vi "Get Analog Vars.vi"(0 "Common alarm handling(F)":bool, 7 "Tool":bool, 11 "error in (no error)":errorcluster) -> (4 "Catagorised  Stsaus":T1[](array[typedef]), 6 "Values":dbl[](array[numeric]), 8 "Analog Vars":T4[](array[typedef]) {"Value" format="%#.1f"}, 10 "Any Alarm":bool, 13 "Primary Action":T3, 14 "Alarms":bool[](array[boolean]), 15 "error out":errorcluster)   [LabVIEW 2011]
uses:
  GUI/Analog Var Disp 0 sif.ctl
  GUI/Status indicator Black Small.ctl
  Action List.ctl
  Catagorised alarm state.ctl
  GUI/Status Indikator Helper.ctl
  Common/Variable List Common Analog.ctl
  Tool/Variable List Tool Analog.ctl
  Action Analog Handler.ctl
  <vilib>/Utility/VariantDataType/GetNumericInfo.vi
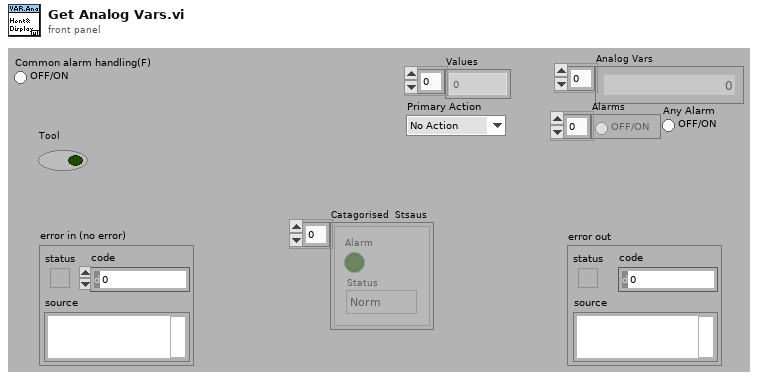
[diagram p1: front panel]
types:
  T1 = typedef "Catagorised alarm state.ctl" = cluster{"Alarm":bool, "Status":T2}
  T2 = typedef "Status Indikator Helper.ctl" = enum16{"Norm", "L", "H", "LL", "HH", "Value", "Technical"}
  T3 = typedef "Action List.ctl" = enum16{"No Action", "Stop Motor", "Turn Off HV"}
  T4 = typedef "Analog Var Disp 0 sif.ctl" = cluster{"Value":dbl, "Unit":string, "Status":T5}
  T5 = typedef "Status indicator Black Small.ctl" = u16
  T6 = typedef "Variable List Tool Analog.ctl" = enum16{"Tool Max Temperature", "Tool (Controller) Temperature", "Tool Supply Voltage", "Tool (Controller) Current", "Tool Acceleration X", "Tool Acceleration Y", "Tool Acceleration Z", "Tool Acceleration Sum", "Tool Inclination", "Tool Rotation", "Tool GP Sensor 1", "Tool GP Sensor 2", "Tool (Pressure 1) Temperature", "Tool Pressure 1 RAW", "Tool (Pressure 2) Temperature", "Tool Pressure 2 RAW", "Tool (Solenoid) Temperature", "Tool Solenoid Position", "PSU Temp", "Head Voltage", "PSU Main Voltage out", "PSU Main Current out", "Upper Tension Sub Temp", "Tool Upper Tension Sub Raw", "Lower Tension Sub Temp", "Tool Lower Tension Sub Raw", "Tool Var27 - Reserved", "Tool Var28 - Reserved", "Tool Var29 - Reserved", "Tool Var30 - Reserved", "Stroke Extension", "Stroke In Force", "Stroke Out Force", "Stroke Force", "Stroker Pressure 1", "Stroker Pressure 2", "Stroker Upper Tension Sub", "Stroker Lower Tension Sub", "Stroker Var09 - Reserved", "Stroker Var10 - Reserved", "Tractor Upper Tension Sub", "Tractor Lower Tension Sub", "Tractor Var03 - Reserved", "Tractor Var04 - Reserved", "Tool Temperature sensor", "Tool Motor Voltage", "Tool Motor Current", "Tool Motor Torque", "Tool weight on bit", "Tool Motor RPM"}
  T7 = typedef "Variable List Common Analog.ctl" = enum16{"HVPSU Head Voltage", "HVPSU TS Voltage", "HVPSU Current", "PCP Cable Resistance", "Winch Depth", "Winch Line Speed", "Winch Wire Tension"}
  T8 = typedef "Action Analog Handler.ctl" = enum16{"GET value", "GET Single Frequenzy", "GET All Values", "GET Waveform", "Get Numb Var", "SET Value", "START Buffer", "REG Variable", "BUF size(total antal sekund)", "PULS", "Get a Value at time", "Set initial waveform"}
  T9 = typedef "User Setting Analog Channel Bg.ctl" = cluster{"Scaling":T10, "Limits and responces":T11, "Allow Graph selection by user":bool, "Unit":u16}
  T10 = typedef "Scaling.ctl" = cluster{"Gain":dbl, "Offset":dbl}
  T11 = typedef "Alarm Setup Analog.ctl" = cluster{"Technical Error(NA)":T12, "LL":T12, "L":T12, "H":T12, "HH":T12, "Limits":T13}
  T12 = typedef "Alarm Responce.ctl" = cluster{"Action":T3, "Alarm":bool}
  T13 = typedef "Limits.ctl" = cluster{"LL":dbl, "L":dbl, "H":dbl, "HH":dbl}
  T14 = typedef "Fixed Analog Channel Definition.ctl" = cluster{"ID":u16, "Name":string, "Quantity":T15, "Unit":string, "Maximum upd":T16, "Comment":string, "Help file Name":string, "Help file Section ":string, "Category":T17, "User adjustable Scaling":bool, "Default Scaling":T10, "Default Unit":i32, "Classification":T18}
  T15 = typedef "Quantity enum.ctl" = enum16{"NA", "Acceleration", "Angle", "Current", "Force", "Distance", "Pressure", "Resistance", "Rotational Speed", "Speed", "Temperature", "Tension", "Torque", "Voltage", "Weight"}
  T16 = typedef "Update frequensies.ctl" = enum16{"2 Hz", "1 Hz", "0.1 Hz"}
  T17 = typedef "Channel catagory Enum.ctl" = enum16{"No Category", "Power", "Temperature", "Pressure"}
  T18 = typedef "Channel Classification Enum.ctl" = enum16{"Basic", "Advanced", "Expert", "Unused"}
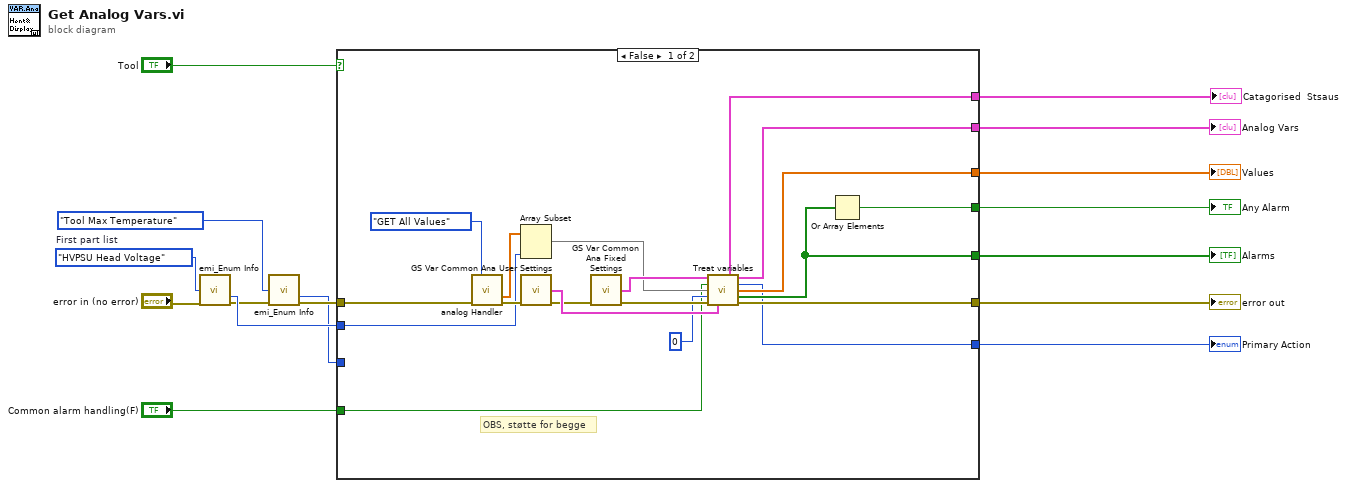
[diagram p0: block diagram]
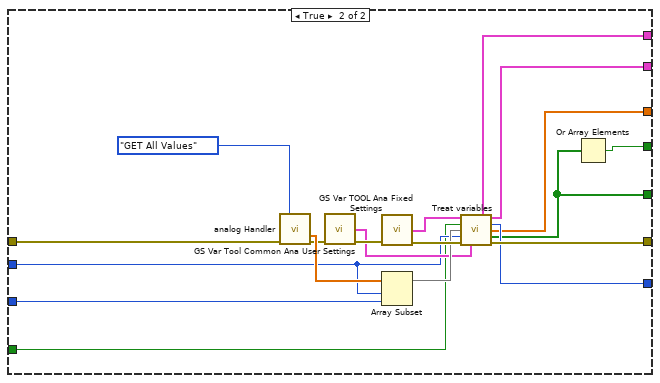
[diagram p2: hidden frame]
diagram:
  w7 = Variable_List_Common_Analog."HVPSU Head Voltage"  # First part list
  n1 = call "emi_Enum Info.vi"("Enum"=w7, "error in (no error)"="error in (no error)") -> ("Numb Elements"=w10:i32, "error out"=w4:errorcluster)  [unwired: 10 in, 2 out]
  n2 = call "emi_Enum Info.vi"("Enum"=Variable_List_Tool_Analog."Tool Max Temperature", "error in (no error)"=w4) -> ("Numb Elements"=w1:i32, "error out"=w3:errorcluster)  [unwired: 10 in, 2 out]
  n3 = case shown="False" "Tool" {
    tunnel: [w29 w39] -> w16
    tunnel: [w28 w42] -> w15
    tunnel: [w27 w41] -> w14
    tunnel: [w26 w45] -> w13
    tunnel: [w25 w40] -> w12
    tunnel: w3 -> [w24 w46]
    tunnel: w10 -> [w21 w44]
    tunnel: [w20 w43] -> w9
    tunnel: [w18 w38] -> w8
    tunnel: "Common alarm handling(F)" -> [w17 w37]
    tunnel: w1 -> [_ w36]
    frame False {
      # "OBS, støtte for begge"
      n4 = call "analog Handler.vi"("Action"=Action_Analog_Handler."GET All Values" ("Action(GET)"), "error in (no error)"=w24) -> ("Values"=w32:dbl[], "error out"=w23:errorcluster)  [unwired: 8 in, 4 out]
      n5 = Array Subset(array=w32, length=w21) -> (w22:dbl[])  [unwired: 1 in]
      n6 = call "GS Var Common Ana User Settings.vi"("error in (no error)"=w23) -> ("Common Analog var User set out"=w33:T9[], "error out"=w30:errorcluster)  [unwired: 12 in, 1 out]
      n7 = call "GS Var Common Ana Fixed Settings.vi"("error in (no error)"=w30) -> ("Common Analog Var Fixed out"=w34:T14[], "error out"=w35:errorcluster)  [unwired: 12 in, 1 out]
      n8 = call "Treat variables.vi"("Analog Variable info fixed"=w34, "Common alarm handling(F)"=w17, "Analog values"=w22, "Variabel start index"=0, "error In"=w35, "Analog Variable info Settings"=w33) -> ("Catagorised  Stsaus"=w18:T1[], "Analog Variable Display"=w29:T4[], "Action"=w20:T3, "Analog Values"=w25:dbl[], "Alarms"=w28:bool[], "error out"=w26:errorcluster)  [unwired: 4 in]
      n9 = Or Array Elements(Boolean array=w28) -> (logical OR=w27:bool)
    }
    frame True {
      n10 = call "analog Handler.vi"("Action"=Action_Analog_Handler."GET All Values" ("Action(GET)"), "error in (no error)"=w46) -> ("Values"=w54:dbl[], "error out"=w52:errorcluster)  [unwired: 8 in, 4 out]
      n11 = call "GS Var Tool Common Ana User Settings.vi"("error in (no error)"=w52) -> ("Tool Analog var User settigns out"=w47:T9[], "error out"=w51:errorcluster)  [unwired: 12 in, 1 out]
      n12 = call "GS Var TOOL Ana Fixed Settings.vi"("error in (no error)"=w51) -> ("Tool Analog var Fixed out"=w49:T14[], "error out"=w50:errorcluster)  [unwired: 12 in, 1 out]
      n13 = Array Subset(array=w54, index=w44, length=w36) -> (w48:dbl[])
      n14 = call "Treat variables.vi"("Analog Variable info fixed"=w49, "Common alarm handling(F)"=w37, "Analog values"=w48, "Variabel start index"=w44, "error In"=w50, "Analog Variable info Settings"=w47) -> ("Catagorised  Stsaus"=w38:T1[], "Analog Variable Display"=w39:T4[], "Action"=w43:T3, "Analog Values"=w40:dbl[], "Alarms"=w42:bool[], "error out"=w45:errorcluster)  [unwired: 4 in]
      n15 = Or Array Elements(Boolean array=w42) -> (logical OR=w41:bool)
    }
  }
  "Analog Vars" <- w16
  "Alarms" <- w15
  "Any Alarm" <- w14
  "error out" <- w13
  "Values" <- w12
  "Primary Action" <- w9
  "Catagorised  Stsaus" <- w8
